vi "Assign Pixel to Wing Sector (FPGA).vi"(6 "Pixel Intensity In":u8, 7 "Right Wing?":bool, 8 "Sector Parameters":T1, 9 "Pixel Y":u16, 10 "Pixel X":u16) -> (1 "Pixel Intensity Out":u8, 2 "sector #":u8, 3 "output valid":bool)   [LabVIEW 2013, in "FPGA Image Processing.lvlib"]
uses:
  FPGA Image Processing.lvlib
  Sector/Accumulate/Sector Parameter Cluster.ctl
  <vilib>/rvi/FXPMathLib/FxpRectToPolar/XNode/nifxpmath_RectToPolar.xnode
  <vilib>/rvi/FXPMathLib/FxpSub/XNode/nifxpmath_Sub.xnode
  <vilib>/rvi/FXPMathLib/sim/FxpSim.dll
  <vilib>/rvi/FXPMathLib/FxpAdd/XNode/nifxpmath_Add.xnode
  <vilib>/rvi/FXPMathLib/FxpDiv/XNode/nifxpmath_Div.xnode
  <vilib>/rvi/FXPMathLib/FxpRectToPolar/simVIs/DllFxpRectToPolarTemp_sub.vi
  <vilib>/rvi/FXPMathLib/FxpRectToPolar/subVIs/nifxpmath_RectToPolar_SimConfig.ctl
  <vilib>/rvi/FXPMathLib/FxpDiv/simVIs/DllFxpDivTemp_sub.vi
  <vilib>/rvi/FXPMathLib/FxpDiv/subVIs/nifxpmath_Div_SimConfig.ctl
  <vilib>/ptbypt/NI_PtbyPt.lvlib
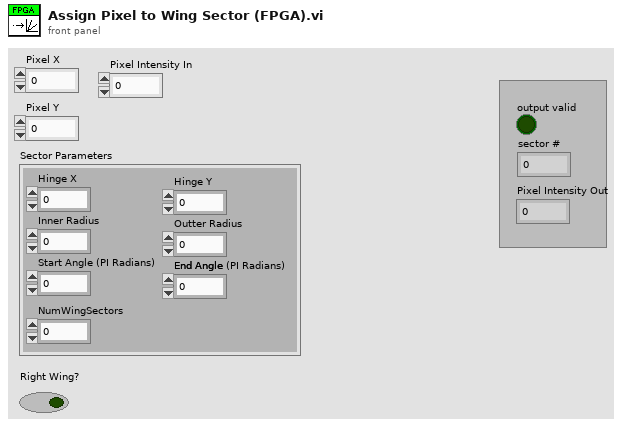
[diagram p1: front panel]
types:
  T1 = typedef "Sector Parameter Cluster.ctl" = cluster{"Start Angle":fxp<+/-,17,2>, "End Angle":fxp<+,17,3>, "Inner Radius":u16, "Outter Radius":u16, "Hinge X":u16, "Hinge Y":u16, "NumWingSectors":u8}
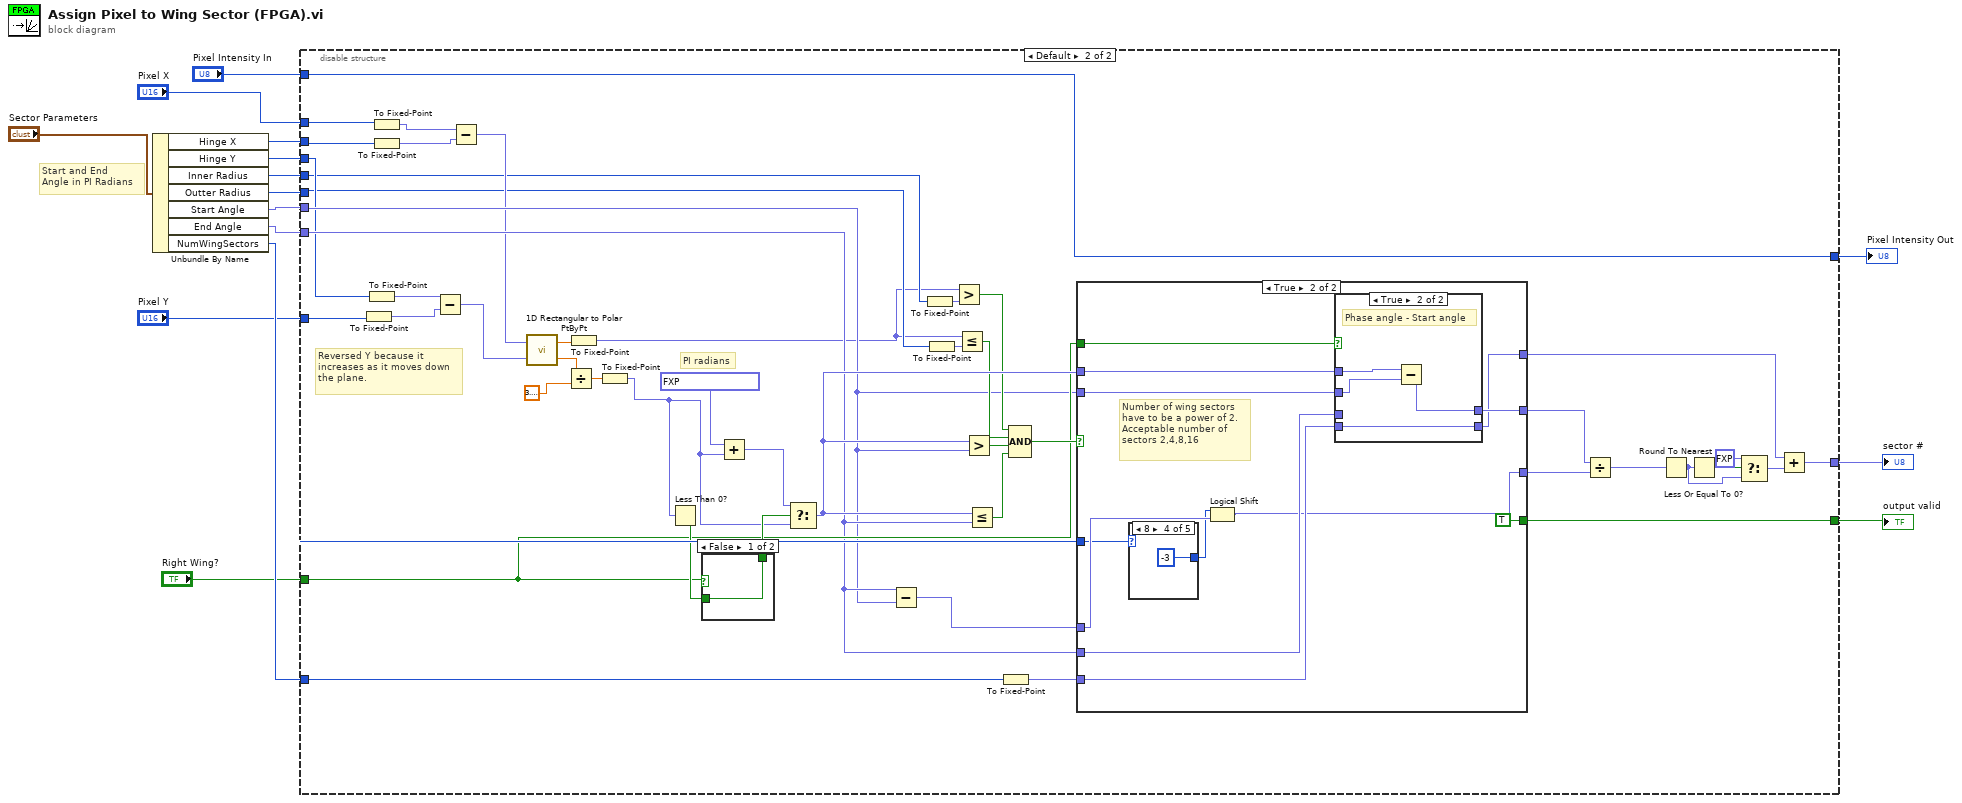
[diagram p0: block diagram]
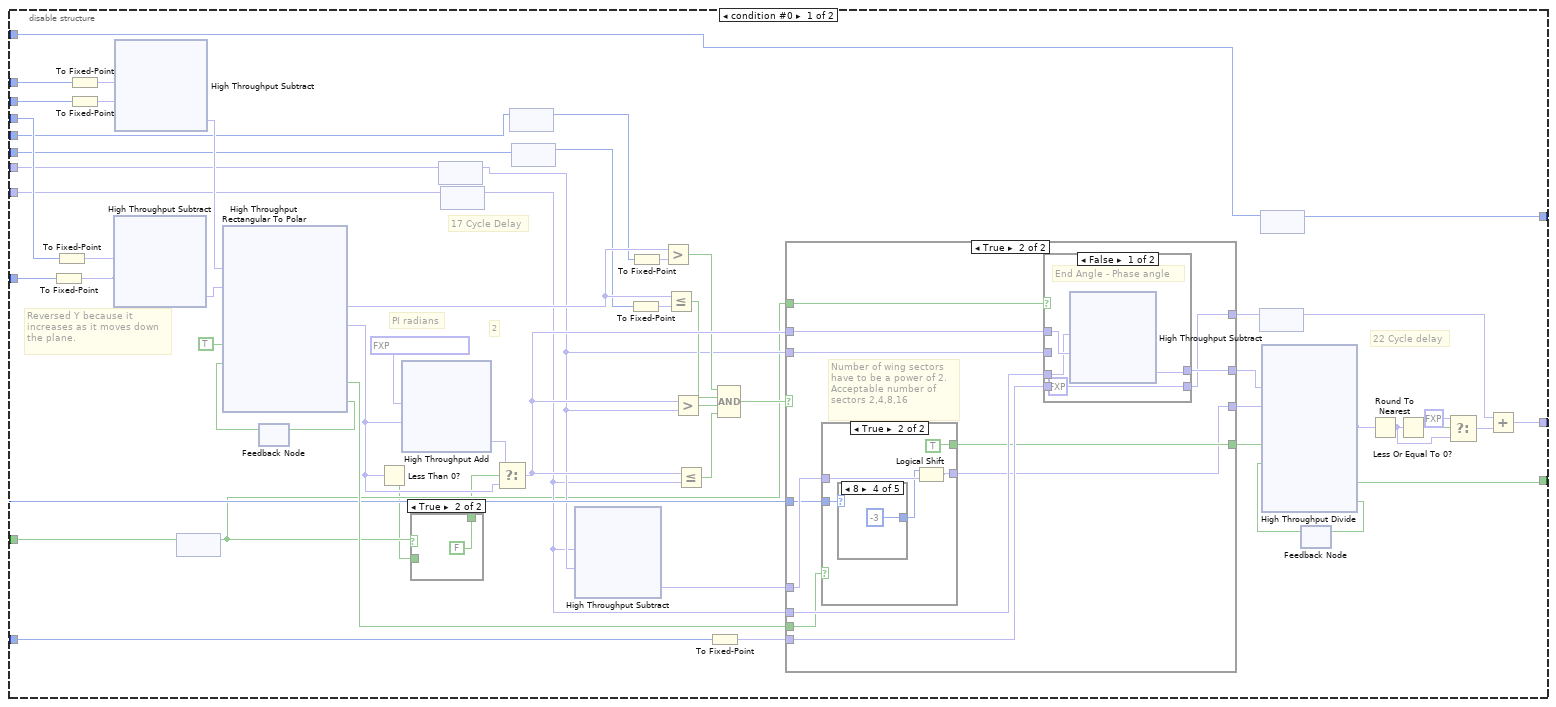
[diagram p2: hidden frame]
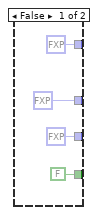
[diagram p4: hidden frame]
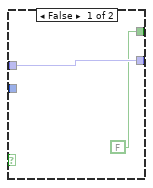
[diagram p5: hidden frame]
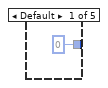
[diagram p6: hidden frame]
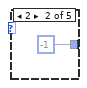
[diagram p7: hidden frame]
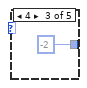
[diagram p8: hidden frame]
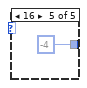
[diagram p9: hidden frame]
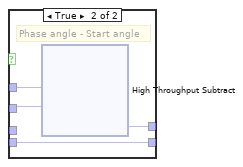
[diagram p10: hidden frame]
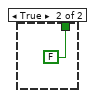
[diagram p11: hidden frame]
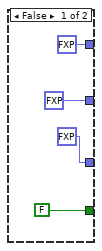
[diagram p12: hidden frame]
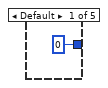
[diagram p13: hidden frame]
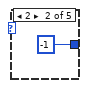
[diagram p14: hidden frame]
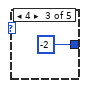
[diagram p15: hidden frame]
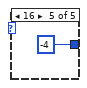
[diagram p16: hidden frame]
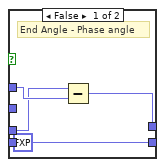
[diagram p17: hidden frame]
diagram:
  # "Start and End\nAngle in PI Radians"
  n1 = Unbundle By Name("Sector Parameters") -> ("Hinge X"=w10:u16, "Hinge Y"=w15:u16, "Inner Radius"=w8:u16, "Outter Radius"=w7:u16, "Start Angle"=w6:fxp<+/-,17,2>, "End Angle"=w5:fxp<+,17,3>, "NumWingSectors"=w14:u8)
  n2 = disable-structure shown="Default" {
    disable-tunnel: w15 -> [w57 w191]
    disable-tunnel: w14 -> [w42 w217]
    disable-tunnel: [w41 w199] -> w13
    disable-tunnel: "Pixel Y" -> [w40 w188]
    disable-tunnel: "Pixel X" -> [w39 w195]
    disable-tunnel: w10 -> [w38 w194]
    disable-tunnel: w8 -> [w37 w187]
    disable-tunnel: w7 -> [w35 w185]
    disable-tunnel: w6 -> [w33 w202]
    disable-tunnel: w5 -> [w31 w203]
    disable-tunnel: [w28 w215] -> w4
    disable-tunnel: "Right Wing?" -> [w18 w205]
    disable-tunnel: "Pixel Intensity In" -> [w17 w199]
    disable-tunnel: [w16 w198] -> w1
    frame condition #0 {
      # "17 Cycle Delay"
      # "Reversed Y because it\nincreases as it moves down\nthe plane."
      # "PI radians"
      # "22 Cycle delay"
      # "2"
      n3 = To Fixed-Point(number=w40) -> (fixed-point=w47:fxp<+,11,11>)  [unwired: 1 in]
      n4 = To Fixed-Point(number=w57) -> (fixed-point=w48:fxp<+,11,11>)  [unwired: 1 in]
      n5 = To Fixed-Point(number=w39) -> (fixed-point=w46:fxp<+,11,11>)  [unwired: 1 in]
      n6 = To Fixed-Point(number=w38) -> (fixed-point=w45:fxp<+,11,11>)  [unwired: 1 in]
      n7 = xnode "High Throughput Subtract"("x"=w48, "y"=w47) -> ("x-y"=w56:fxp<+/-,12,12>)
      n8 = xnode "High Throughput Subtract"("x"=w46, "y"=w45) -> ("x-y"=w55:fxp<+/-,12,12>)
      n9 = feedback #1() -> (w27:bool)  [unwired: 1 in]
      n10 = feedback-in #1(w18) -> ()
      n11 = feedback #2() -> (w62:bool)  [unwired: 1 in]
      n12 = xnode "High Throughput Rectangular To Polar"("x"=w55, "y"=w56, "input valid"=TRUE, "ready for output (T)"=w62) -> ("magnitude"=w71:fxp<+,12,12>, "phase (pi)"=w68:fxp<+/-,16,2>, "output valid"=w43:bool, "ready for input"=w63:bool)
      n13 = feedback-in #2(w63) -> ()
      n14 = Less Than 0?(x=w68) -> (x < 0?=w25:bool)
      n15 = xnode ("High Throughput Add")("x"=fxp<+/-,16,2> 1.99993896484375 ("y"), "y"=w68) -> ("x+y"=w67:fxp<+/-,17,3>)
      n16 = case shown="True" w27 {
        tunnel: [w73 FALSE ("s")] -> w26
        tunnel: w25 -> [w73 _]
        frame False {
        }
        frame True {
        }
      }
      n17 = feedback #3() -> (w32:fxp<+/-,17,2>)  [unwired: 1 in]
      n18 = feedback-in #3(w33) -> ()
      n19 = feedback #4() -> (w30:fxp<+,17,3>)  [unwired: 1 in]
      n20 = feedback-in #4(w31) -> ()
      n21 = Select(t=w67, s=w26, f=w68) -> (s? t:f=w65:fxp<+/-,17,3>)
      n22 = feedback #5() -> (w36:u16)  [unwired: 1 in]
      n23 = feedback-in #5(w37) -> ()
      n24 = feedback #6() -> (w34:u16)  [unwired: 1 in]
      n25 = feedback-in #6(w35) -> ()
      n26 = xnode ("High Throughput Subtract")("x"=w30, "y"=w32) -> ("x-y"=w44:fxp<+/-,17,6>)
      n27 = To Fixed-Point(number=w34) -> (fixed-point=w70:fxp<+,16,16>)  [unwired: 1 in]
      n28 = To Fixed-Point(number=w36) -> (fixed-point=w72:fxp<+,16,16>)  [unwired: 1 in]
      n29 = Greater?(x=w71, y=w72) -> (0:w61:bool)
      n30 = Less Or Equal?(x=w71, y=w70) -> (x <= y?=w60:bool)
      n31 = Greater?(x=w65, y=w32) -> (0:w59:bool)
      n32 = Less Or Equal?(x=w65, y=w30) -> (x <= y?=w58:bool)
      n33 = To Fixed-Point(number=w42) -> (fixed-point=w24:fxp<+,8,8>)  [unwired: 1 in]
      n34 = Compound Arithmetic op=AND(w61, w60, w59, w58) -> (w69:bool)
      n35 = case shown="True" w69 {
        tunnel: w65 -> [_ w119]
        tunnel: w32 -> [_ w118]
        tunnel: [fxp<+/-,17,6> 0.0 ("x-y") w109] -> w52
        tunnel: w30 -> [_ w116]
        tunnel: w24 -> [_ w117]
        tunnel: [fxp<+/-,20,5> 0.0 ("x-y") w115] -> w53
        tunnel: [FALSE ("output valid") w110] -> w51
        tunnel: [fxp<+,8,8> 0.0 w114] -> w49
        tunnel: w44 -> [_ w113]
        tunnel: w43 -> [_ w112]
        tunnel: w42 -> [_ w111]
        tunnel: w27 -> [_ w108]
        frame False {
        }
        frame True {
          # "Number of wing sectors\nhave to be a power of 2.\nAcceptable number of\nsectors 2,4,8,16"
          n36 = case shown="True" w112 {
            tunnel: w111 -> [_ w126]
            tunnel: w113 -> [w121 w125]
            tunnel: [w121 w123] -> w109
            tunnel: [FALSE ("output valid") TRUE ("output valid")] -> w110
            frame False {
            }
            frame True {
              n37 = case shown="8" w126 {
                tunnel: [i16 0 ("y") i16 -1 ("y") i16 -2 ("y") i16 -3 ("y") i16 -4 ("y")] -> w124
                frame Default {
                }
                frame 2 {
                }
                frame 4 {
                }
                frame 8 {
                }
                frame 16 {
                }
              }
              n38 = Logical Shift(y=w124, x=w125) -> (x << y=w123:fxp<+/-,17,6>)
            }
          }
          n39 = case shown="False" w108 {
            tunnel: w119 -> [w134 w139]
            tunnel: w118 -> [_ w138]
            tunnel: [w135 w137] -> w115
            tunnel: w117 -> [_ w136]
            tunnel: [fxp<+,8,8> 0.0 w136] -> w114
            tunnel: w116 -> [w133 _]
            frame False {
              # "End Angle - Phase angle"
              n40 = xnode "High Throughput Subtract"("x"=w133, "y"=w134) -> ("x-y"=w135:fxp<+/-,19,5>)
            }
            frame True {
              # "Phase angle - Start angle"
              n41 = xnode ("High Throughput Subtract")("x"=w139, "y"=w138) -> ("x-y"=w137:fxp<+/-,19,4>)
            }
          }
        }
      }
      n42 = feedback #7() -> (w19:fxp<+,8,8>)  [unwired: 1 in]
      n43 = feedback-in #7(w49) -> ()
      n44 = feedback #8() -> (w41:u8)  [unwired: 1 in]
      n45 = feedback-in #8(w17) -> ()
      n46 = feedback #9() -> (w50:bool)  [unwired: 1 in]
      n47 = xnode "High Throughput Divide"("x"=w53, "y"=w52, "input valid"=w51, "ready for output (T)"=w50) -> ("x/y"=w21:fxp<+/-,20,16>, "output valid"=w16:bool, "ready for input"=w54:bool)
      n48 = feedback-in #9(w54) -> ()
      n49 = Round To Nearest(number=w21) -> (nearest integer value=w20:fxp<+/-,17,17>)
      n50 = Less Or Equal To 0?(x=w20) -> (x <= 0?=w23:bool)
      n51 = Select(t=fxp<+/-,17,17> 1.0, s=w23, f=w20) -> (s? t:f=w29:fxp<+/-,17,17>)
      n52 = Add(x=w19, y=w29) -> (x+y=w28:fxp<+/-,17,17>)
    }
    frame condition #1 (active) {
      # "Reversed Y because it\nincreases as it moves down\nthe plane."
      # "PI radians"
      n53 = To Fixed-Point(number=w188) -> (fixed-point=w189:fxp<+,11,11>)  [unwired: 1 in]
      n54 = To Fixed-Point(number=w191) -> (fixed-point=w190:fxp<+,11,11>)  [unwired: 1 in]
      n55 = To Fixed-Point(number=w195) -> (fixed-point=w193:fxp<+,11,11>)  [unwired: 1 in]
      n56 = To Fixed-Point(number=w194) -> (fixed-point=w192:fxp<+,11,11>)  [unwired: 1 in]
      n57 = Subtract(x=w190, y=w189) -> (x-y=w207:fxp<+/-,12,12>)
      n58 = Subtract(x=w193, y=w192) -> (x-y=w196:fxp<+/-,12,12>)
      n59 = call <vilib>:"1D Rectangular to Polar PtByPt.vi"("y"=w207, "x"=w196) -> ("phase"=w206:dbl, "magnitude"=w181:dbl)
      n60 = Divide(x=w206, y=3.141592653589793) -> (x/y=w183:dbl)
      n61 = To Fixed-Point(number=w181) -> (fixed-point=w180:fxp<+,12,12>)  [unwired: 1 in]
      n62 = To Fixed-Point(number=w183) -> (fixed-point=w182:fxp<+/-,16,2>)  [unwired: 1 in]
      n63 = Less Than 0?(x=w182) -> (x < 0?=w213:bool)
      n64 = case shown="False" w205 {
        tunnel: [w226 FALSE ("s")] -> w214
        tunnel: w213 -> [w226 _]
        frame False {
        }
        frame True {
        }
      }
      n65 = Add(x=fxp<+/-,16,2> 1.99993896484375 ("y"), y=w182) -> (x+y=w204:fxp<+/-,17,3>)
      n66 = Select(t=w204, s=w214, f=w182) -> (s? t:f=w224:fxp<+/-,17,3>)
      n67 = Subtract(x=w203, y=w202) -> (x-y=w201:fxp<+/-,20,5>)
      n68 = To Fixed-Point(number=w187) -> (fixed-point=w186:fxp<+,16,16>)  [unwired: 1 in]
      n69 = To Fixed-Point(number=w185) -> (fixed-point=w184:fxp<+,16,16>)  [unwired: 1 in]
      n70 = Greater?(x=w180, y=w186) -> (0:w223:bool)
      n71 = Less Or Equal?(x=w180, y=w184) -> (x <= y?=w222:bool)
      n72 = Greater?(x=w224, y=w202) -> (0:w221:bool)
      n73 = Less Or Equal?(x=w224, y=w203) -> (x <= y?=w220:bool)
      n74 = To Fixed-Point(number=w217) -> (fixed-point=w212:fxp<+,8,8>)  [unwired: 1 in]
      n75 = Compound Arithmetic op=AND(w223, w222, w221, w220) -> (w225:bool)
      n76 = case shown="True" w225 {
        tunnel: w224 -> [_ w243]
        tunnel: w202 -> [_ w242]
        tunnel: [fxp<+/-,17,6> 0.0 ("x-y") w235] -> w218
        tunnel: w203 -> [_ w240]
        tunnel: w212 -> [_ w241]
        tunnel: [fxp<+/-,20,5> 0.0 ("x-y") w239] -> w219
        tunnel: [fxp<+,8,8> 0.0 w238] -> w200
        tunnel: w201 -> [_ w237]
        tunnel: w217 -> [_ w236]
        tunnel: w205 -> [_ w234]
        tunnel: [FALSE ("output valid") TRUE ("output valid")] -> w198
        frame False {
        }
        frame True {
          # "Number of wing sectors\nhave to be a power of 2.\nAcceptable number of\nsectors 2,4,8,16"
          n77 = case shown="8" w236 {
            tunnel: [i16 0 ("y") i16 -1 ("y") i16 -2 ("y") i16 -3 ("y") i16 -4 ("y")] -> w233
            frame Default {
            }
            frame 2 {
            }
            frame 4 {
            }
            frame 8 {
            }
            frame 16 {
            }
          }
          n78 = Logical Shift(y=w233, x=w237) -> (x << y=w235:fxp<+/-,20,5>)
          n79 = case shown="True" w234 {
            tunnel: w243 -> [w251 w256]
            tunnel: w242 -> [_ w255]
            tunnel: [w252 w254] -> w239
            tunnel: w241 -> [_ w253]
            tunnel: [fxp<+,8,8> 0.0 w253] -> w238
            tunnel: w240 -> [w250 _]
            frame False {
              # "End Angle - Phase angle"
              n80 = Subtract(x=w250, y=w251) -> (x-y=w252:fxp<+/-,19,5>)
            }
            frame True {
              # "Phase angle - Start angle"
              n81 = Subtract(x=w256, y=w255) -> (x-y=w254:fxp<+/-,19,4>)
            }
          }
        }
      }
      n82 = Divide(x=w219, y=w218) -> (x/y=w209:fxp<+/-,20,16>)
      n83 = Round To Nearest(number=w209) -> (nearest integer value=w208:fxp<+/-,17,17>)
      n84 = Less Or Equal To 0?(x=w208) -> (x <= 0?=w211:bool)
      n85 = Select(t=fxp<+/-,17,17> 1.0, s=w211, f=w208) -> (s? t:f=w216:fxp<+/-,17,17>)
      n86 = Add(x=w200, y=w216) -> (x+y=w215:fxp<+/-,17,17>)
    }
  }
  "output valid" <- w1
  "Pixel Intensity Out" <- w13
  "sector #" <- w4
